vi "20211224_01.vi"(1 "Side C":string="0" caption="Side C(C邊)", 2 "Side B":string="0" caption="Side B(B邊)", 3 "Side A":string="0" caption="Side A(A邊)") -> (0 "Area":dbl caption="Area(面積)")   [LabVIEW 2019]
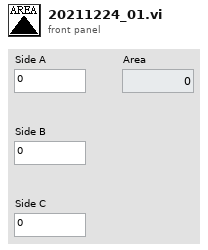
[diagram p1: front panel]
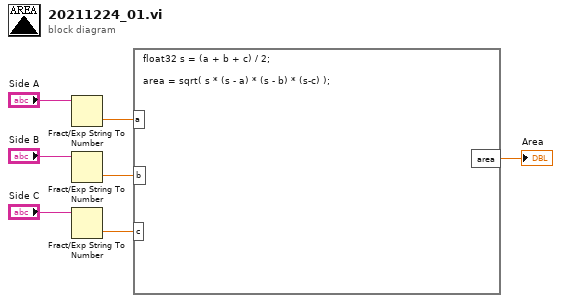
[diagram p0: block diagram]
diagram:
  n1 = Fract/Exp String To Number(string="Side A") -> (number=w5:dbl)  [unwired: 3 in, 1 out]
  n2 = Fract/Exp String To Number(string="Side B") -> (number=w3:dbl)  [unwired: 3 in, 1 out]
  n3 = Fract/Exp String To Number(string="Side C") -> (number=w1:dbl)  [unwired: 3 in, 1 out]
  n4 = formula code="float32 s = (a + b + c) / 2;\n\narea = sqrt( s * (s - a) * (s - b) * (s-c) );"("a"=w5, "b"=w3, "c"=w1) -> ("area"=→"Area":dbl)
